vi "theta_vec2array.vi"(2 "error in (no error)":errorcluster, 3 "Real Matrix":T1) -> (0 "error out":errorcluster, 1 "appended array":dbl[](array[numeric]))   [LabVIEW 2021]
uses:
  <vilib>/Analysis/Matrix/Datatypes/RealMatrix.ctl
  <vilib>/Analysis/Matrix/NI_Matrix.lvlib
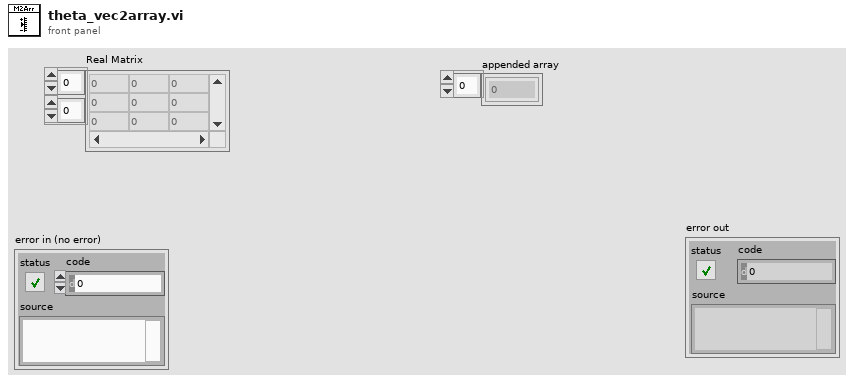
[diagram p1: front panel]
types:
  T1 = typedef "NI_Matrix.lvlib/RealMatrix.ctl" = dbl[][]
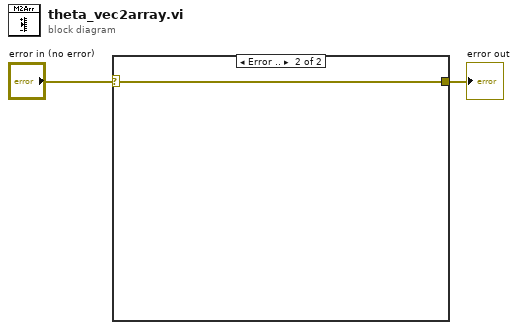
[diagram p0: block diagram]
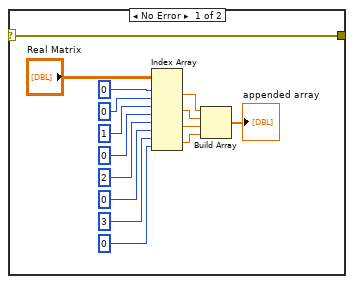
[diagram p2: hidden frame]
diagram:
  n1 = case shown="Error .." "error in (no error)" {
    selector: "error in (no error)" -> [w17 w18]
    tunnel: [w17 w18] -> w1
    frame No Error {
      n2 = Index Array(array="Real Matrix", index (row) #1=0 ("index (row)"), index (col) #1=0 ("index (col)"), index (row) #2=1 ("index (row)"), index (col) #2=0 ("index (col)"), index (row) #3=2 ("index (row)"), index (col) #3=0 ("index (col)"), index (row) #4=3 ("index (row)"), index (col) #4=0 ("index (col)")) -> (element #1=w7:dbl, element #2=w6:dbl, element #3=w5:dbl, element #4=w4:dbl)
      n3 = Build Array(w7, w6, w5, w4) -> (→"appended array":dbl[])
    }
    frame Error {
    }
  }
  "error out" <- w1
